vi "VI Scripting with Structures - Case Structure.vi"   [LabVIEW 2019]
doc: "This example contains sample code demonstrating common VI Scripting navigational tasks relating to Case Structures."
panel:
  # "Overview: Illustrates several CaseStructure properties and methods used for inspecting and modifying Case Structures with VI Scripting.\nInstructions:\nOpen the block diagram of this VI to see several examples of properties and methods related to Case Structures and VI Scripting.\n\nNote: Browse the diagram of this example to learn about VI Scripting concepts. This example is not meant to be run."
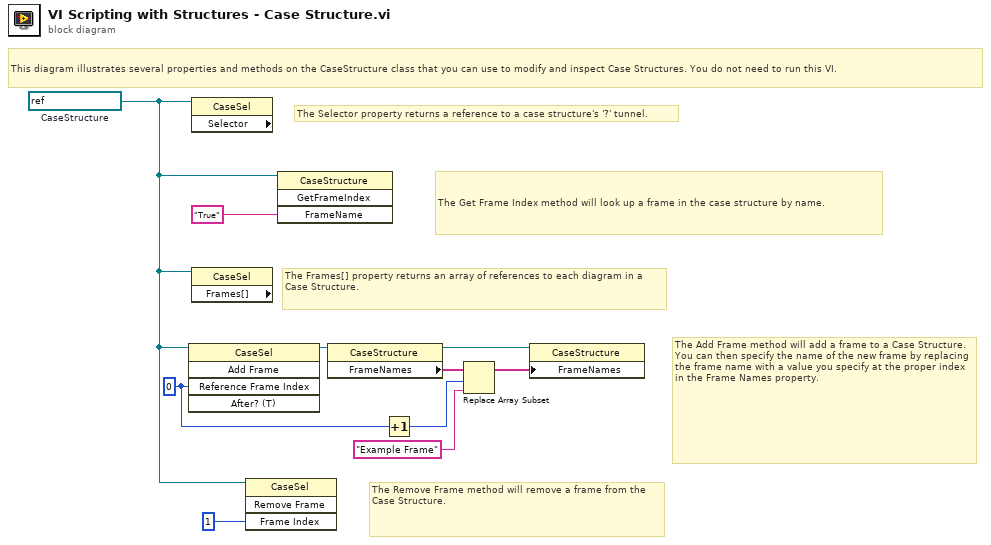
[diagram p0: block diagram]
diagram:
  w4 = u32 0 ("Reference Frame Index")
  w2 = refnum<vi> refnum  # CaseStructure
  # "This diagram illustrates several properties and methods on the CaseStructure class that you can use to modify and inspect Case Structures. You do not need to run this VI."
  # "The Remove Frame method will remove a frame from the Case Structure."
  # "The Add Frame method will add a frame to a Case Structure. You can then specify the name of the new frame by replacing the frame name with a value you specify at the proper index in the Frame Names property."
  # "The Frames[] property returns an array of references to each diagram in a Case Structure."
  # "The Get Frame Index method will look up a frame in the case structure by name."
  # "The Selector property returns a reference to a case structure's '?' tunnel."
  n1 = invoke class="CaseSel" method="Add Frame"(reference=w2, "Reference Frame Index"=w4) -> (reference out=w9:refnum<vi>)  [unwired: 3 in, 4 out]
  n2 = property class="CaseSel" props=["Selector"](reference=w2) -> ()  [unwired: 1 in, 3 out]
  n3 = property class="CaseSel" props=["Frames[]"](reference=w2) -> ()  [unwired: 1 in, 3 out]
  n4 = invoke class="CaseSel" method="Remove Frame"(reference=w2, "Frame Index"=u32 1) -> ()  [unwired: 2 in, 4 out]
  n5 = invoke class="CaseStructure" method="GetFrameIndex"(reference=w2, "FrameName"="True" ("Frame Name")) -> ()  [unwired: 2 in, 4 out]
  n6 = property class="CaseStructure"(reference=w9) -> (reference out=w7:refnum<vi>, "FrameNames"=w8:string[])  [unwired: 1 in, 1 out]
  n7 = Increment(x=w4) -> (x+1=w5:u32)
  n8 = Replace Array Subset(array=w8, new element="Example Frame" ("new element/subarray"), index=w5) -> (w6:string[])
  n9 = property class="CaseStructure"(reference=w7, "FrameNames"=w6) -> ()  [unwired: 1 in, 2 out]
